vi "Begin.vi"(11 "Image Size":T1=enum."160x120") -> (0 "error out":errorcluster)   [LabVIEW 2012]
doc: "Called before other user functions, this VI is expected to open initial I/O refnums, load in file data, and do all program initialization. Notice that the <B>error out</B> terminal is simply used for data flow. Wiring it to other structures or subVIs ensures that this VI runs first."
uses:
  <vilib>/Rock Robotics/WPI/Camera/WPI_CameraImageSize.ctl
  <vilib>/Rock Robotics/SystemInterfaces/DIO/FPGA_DIOPWMChannel.ctl
  <vilib>/Rock Robotics/WPI/Camera/WPI_CameraWhite Balance Values.ctl
  <vilib>/Rock Robotics/WPI/Camera/WPI_CameraExposure Values.ctl
  <vilib>/Rock Robotics/WPI/Camera/WPI_CameraFrameRate.ctl
  <vilib>/Rock Robotics/WPI/SafetyOutput/WPI_SafetyOutputConfigMenu.ctl
  <vilib>/Rock Robotics/WPI/DriverStation/WPI_DriverStationRobotMode2.ctl
  <vilib>/Rock Robotics/WPI/Joystick/WPI_JoystickDeviceEnum.ctl
  <vilib>/Rock Robotics/WPI/Solenoid/WPI_SolenoidChannel.ctl
  <vilib>/Rock Robotics/SystemInterfaces/DIO/FPGA_DIOChannel.ctl
  <vilib>/Rock Robotics/SystemInterfaces/DIO/FPGA_DIORelayChannel.ctl
  <vilib>/Rock Robotics/SystemInterfaces/Typedef/FPGA_TypedefSolenoidModule.ctl
  <vilib>/Rock Robotics/SystemInterfaces/Typedef/FPGA_TypedefDigitalModule.ctl
  Robot Global Data.vi
  <vilib>/Rock Robotics/WPI/MotorControl/WPI_MotorControlOpen Talon.vi
  <vilib>/Rock Robotics/WPI/RobotDrive/WPI_RobotDriveOpen4MotorWithTalon.vi
  <vilib>/Rock Robotics/WPI/Solenoid/WPI_SolenoidOpenSingle.vi
  <vilib>/Rock Robotics/WPI/Compressor/WPI_CompressorGetSetRefNum.vi
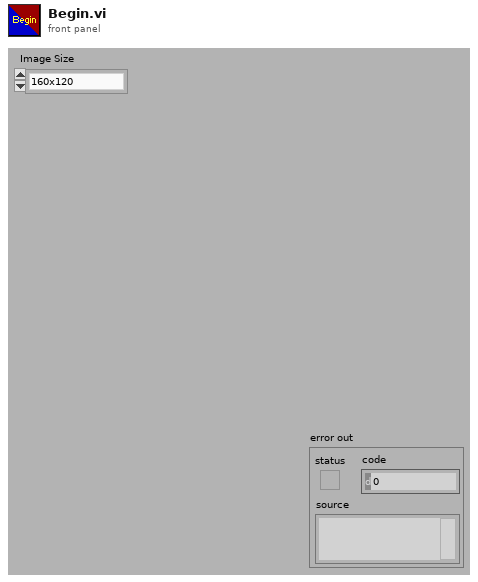
[diagram p1: front panel]
types:
  T1 = typedef "WPI_CameraImageSize.ctl" = enum16{"640x480", "320x240", "160x120"}
  T2 = typedef "WPI_SolenoidChannel.ctl" = enum8{"Solenoid 1", "Solenoid 2", "Solenoid 3", "Solenoid 4", "Solenoid 5", "Solenoid 6", "Solenoid 7", "Solenoid 8", "Invalid"}
  T3 = typedef "FPGA_TypedefSolenoidModule.ctl" = enum16{"Solenoid Module 1", "Solenoid Module 2"}
  T4 = typedef "FPGA_DIOChannel.ctl" = enum8{"DIO 1", "DIO 2", "DIO 3", "DIO 4", "DIO 5", "DIO 6", "DIO 7", "DIO 8", "DIO 9", "DIO 10", "DIO 11", "DIO 12", "DIO 13", "DIO 14", "Invalid"}
  T5 = typedef "FPGA_TypedefDigitalModule.ctl" = enum16{"Digital Module 1", "Digital Module 2"}
  T6 = typedef "FPGA_DIORelayChannel.ctl" = enum8{"Relay 1", "Relay 2", "Relay 3", "Relay 4", "Relay 5", "Relay 6", "Relay 7", "Relay 8", "Invalid"}
  T7 = typedef "FPGA_DIOPWMChannel.ctl" = enum8{"PWM 1", "PWM 2", "PWM 3", "PWM 4", "PWM 5", "PWM 6", "PWM 7", "PWM 8", "PWM 9", "PWM 10", "Invalid"}
  T8 = typedef "WPI_SafetyOutputConfigMenu.ctl" = enum16{"Enable", "Disable"}
  T9 = typedef "WPI_JoystickDeviceEnum.ctl" = enum16{"USB 1", "USB 2", "USB 3", "USB 4", "Kinect 1", "Kinect 2"}
  T10 = typedef "WPI_DriverStationRobotMode2.ctl" = enum16{"Autonomous Disabled", "Autonomous Enabled", "Teleop Disabled", "Teleop Enabled", "Timeout", "Finish", "Test Disabled", "Test Enabled"}
  T11 = typedef "WPI_CameraFrameRate.ctl" = u32
  T12 = typedef "WPI_CameraExposure Values.ctl" = enum16{"Auto", "Flicker-free 50 Hz", "Flicker-free 60 Hz", "Hold current"}
  T13 = typedef "WPI_CameraWhite Balance Values.ctl" = enum16{"Auto", "Fixed indoor", "Fixed outdoor 1", "Fixed outdoor 2", "Fixed fluorescent 1", "Fixed fluorescent 2", "Hold current"}
  T14 = typedef "WPI_DigitalOutputDevRef.ctl" = cluster{"Digital Module":T5, "DIO Channel":T4, "DevStatus":errorcluster}
  T15 = typedef "WPI_CompressorDevRef.ctl" = cluster{"DevStatus":errorcluster, "DigitalInputDevRef":T16, "RelayDevRef":T17}
  T16 = typedef "WPI_DigitalInputDevRef.ctl" = cluster{"DevStatus":errorcluster, "DIO Channel":T4, "Digital Module":T5}
  T17 = typedef "WPI_RelayDevRef.ctl" = cluster{"DevStatus":errorcluster, "Relay Channel":T6, "Digital Module":T5, "Relay Direction":T18}
  T18 = typedef "WPI_RelayDirection.ctl" = enum16{"Both directions", "Forward only", "Reverse only"}
  T19 = typedef "WPI_SolenoidDevRef.ctl" = cluster{"DevStatus":errorcluster, "Solenoid Module":T3, "Forward Solenoid Channel":T2, "Reverse Solenoid Channel":T2}
  T20 = typedef "WPI_CameraDevRef.ctl" = cluster{"Camera Address":string, "CameraStatus":errorcluster, "Acquire Image Notifier":refnum<notifier>}
  T21 = typedef "WPI_RobotDriveDevRef.ctl" = cluster{"DevStatus":errorcluster, "Motors[]":T22[], "Square Inputs":bool, "Max Output":dbl, "Isochronous":bool}
  T22 = typedef "WPI_MotorControlDeviceRef.ctl" = cluster{"DeviceStatus":errorcluster, "Type":enum16{"PWM", "CAN"}, "PWM":cluster{"Digital Module":T5, "PWM Channel":T7, "DeadBand":T23}, "CAN":cluster{"Device Number":u8, "Control Mode":T24, "Semaphore":T25, "Max Vout":dbl}, "Invert":bool, "TransformRef":T26, "InvTransformRef":T26}
  T23 = typedef "WPI_PWMDeadband.ctl" = cluster{"Name":string, "maxPositivePwm":i32, "minPositivePwm":i32, "centerPwm":i32, "maxNegativePwm":i32, "minNegativePwm":i32, "angularRange":u16}
  T24 = typedef "WPI_CANJaguar_ControlMode.ctl" = enum8{"Percent VBus", "Current", "Speed", "Position", "Voltage"}
  T25 = typedef "Semaphore RefNum" = refnum<k1>
  T26 = typedef "WPI_PWMTransform_ConPane.ctl" = refnum<vi>
  T27 = typedef "WPI_JoystickDevRef.ctl" = cluster{"Device":T9}
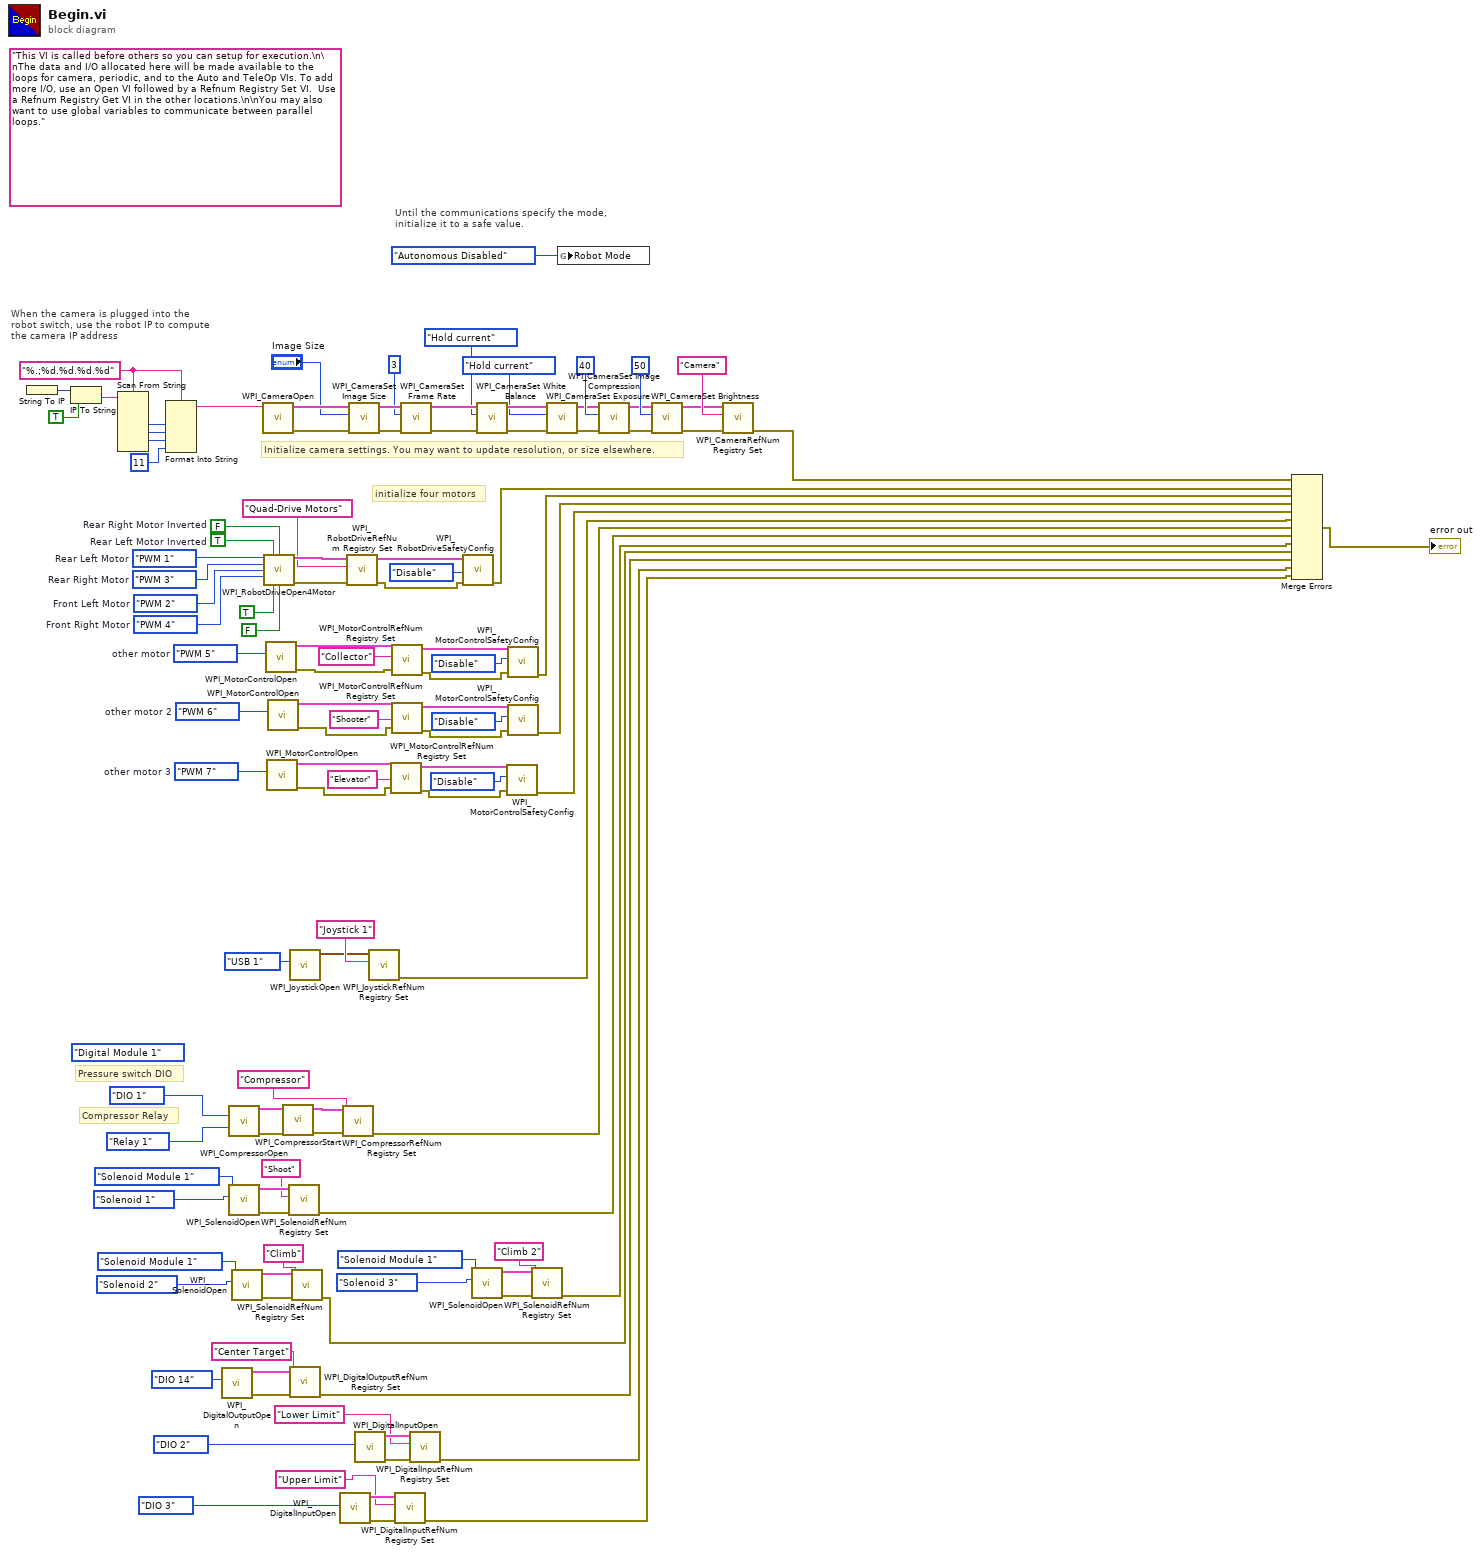
[diagram p0: block diagram]
diagram:
  (unwired) FPGA_TypedefDigitalModule."Digital Module 1" ("Pressure Switch Digital Module (Module 1)")
  w57 = FPGA_DIOPWMChannel."PWM 7"  # other motor 3
  w65 = FPGA_DIOPWMChannel."PWM 6"  # other motor 2
  w69 = FPGA_DIOPWMChannel."PWM 5"  # other motor
  w73 = FPGA_DIOPWMChannel."PWM 4"  # Front Right Motor
  w74 = FPGA_DIOPWMChannel."PWM 2"  # Front Left Motor
  w82 = "%.;%d.%d.%d.%d" ("format string")
  (unwired) "This VI is called before others so you can setup for execution.\n\nThe data and I/O allocated here will be made available to the loops for camera, periodic, and to the Auto and TeleOp VIs. To add more I/O, use an Open VI followed by a Refnum Registry Set VI.  Use a Refnum Registry Get VI in the other locations.\n\nYou may also want to use global variables to communicate between parallel loops."
  w93 = FPGA_DIOPWMChannel."PWM 3"  # Rear Right Motor
  w94 = FPGA_DIOPWMChannel."PWM 1"  # Rear Left Motor
  w116 = TRUE  # Rear Left Motor Inverted
  w117 = FALSE  # Rear Right Motor Inverted
  # "Compressor Relay"
  # "Pressure switch DIO"
  # "Until the communications specify the mode,\ninitialize it to a safe value."
  # "When the camera is plugged into the\nrobot switch, use the robot IP to compute\nthe camera IP address"
  # "initialize four motors"
  # "Initialize camera settings. You may want to update resolution, or size elsewhere."
  n1 = String To IP() -> (0:w89:u32)  [unwired: 1 in]
  n2 = IP To String(1:TRUE ("dot notation? (F)"), 2:w89) -> (0:w87:string)
  n3 = Scan From String(format string=w82, input string=w87) -> (output 1=w86:i32, output 2=w85:i32, output 3=w84:i32)  [unwired: 7 in, 3 out]
  n4 = Format Into String(format string=w82, w86, w85, w84, 11 ("Compression")) -> (resulting string=w78:string)  [unwired: 2 in, 1 out]
  n5 = call <vilib>:"WPI_DigitalOutputOpen.vi"("DIO Channel"=FPGA_DIOChannel."DIO 14") -> ("error out"=w40:errorcluster, "DigitalOutputDevRef"=w50:T14)  [unwired: 9 in]
  n6 = call <vilib>:"WPI_CompressorOpen.vi"("Pressure Switch DIO Channel"=FPGA_DIOChannel."DIO 1", "Relay Channel"=FPGA_DIORelayChannel."Relay 1") -> ("CompressorDevRef"=w36:T15, "error out"=w34:errorcluster)  [unwired: 12 in]
  n7 = call-poly <vilib>:"WPI_SolenoidOpen.vi"("Solenoid Channel"=WPI_SolenoidChannel."Solenoid 1", "Solenoid Module (Module 1)"=FPGA_TypedefSolenoidModule."Solenoid Module 1") -> ("error out"=w41:errorcluster, "SolenoidDevRef"=w53:T19)  [unwired: 8 in]
  n8 = call-poly <vilib>:"WPI_SolenoidOpen.vi"("Solenoid Channel"=WPI_SolenoidChannel."Solenoid 2", "Solenoid Module (Module 1)"=FPGA_TypedefSolenoidModule."Solenoid Module 1") -> ("error out"=w20:errorcluster, "SolenoidDevRef"=w22:T19)  [unwired: 8 in]
  n9 = call <vilib>:"WPI_CameraOpen.vi"("Camera Address"=w78) -> ("error out"=w103:errorcluster, "CameraDevRef"=w104:T20)  [unwired: 2 in, 7 out]
  n10 = call-poly <vilib>:"WPI_RobotDriveOpen4Motor.vi"("Rear Left Motor"=w94, "Rear Left Motor Inverted"=w116, "Rear Right Motor Inverted"=w117, "Rear Right Motor"=w93, "Front Left Motor"=w74, "Front Right Motor"=w73, "Front Left Motor Inverted"=TRUE, "Front Right Motor Inverted"=FALSE) -> ("RobotDriveDevRef"=w114:T21, "error out"=w112:errorcluster)  [unwired: 6 in]
  n11 = call-poly <vilib>:"WPI_MotorControlOpen.vi"("PWM Channel"=w69) -> ("error out"=w46:errorcluster, "MotorControlDeviceRef"=w72:T22)  [unwired: 9 in]
  n12 = call-poly <vilib>:"WPI_MotorControlOpen.vi"("PWM Channel"=w57) -> ("error out"=w42:errorcluster, "MotorControlDeviceRef"=w60:T22)  [unwired: 9 in]
  n13 = call-poly <vilib>:"WPI_MotorControlOpen.vi"("PWM Channel"=w65) -> ("error out"=w45:errorcluster, "MotorControlDeviceRef"=w68:T22)  [unwired: 9 in]
  n14 = call <vilib>:"WPI_CompressorStart.vi"("error in (no error)"=w34, "CompressorDevRef"=w36) -> ("error out"=w33:errorcluster, "CompressorDevRef"=w35:T15)  [unwired: 8 in]
  n15 = call <vilib>:"WPI_SolenoidRefNum Registry Set.vi"("error in (no error)"=w41, "refnum name"="Shoot", "SolenoidDevRef"=w53) -> ("error out"=w8:errorcluster)  [unwired: 7 in, 1 out]
  n16 = call <vilib>:"WPI_JoystickOpen.vi"("JoystickDevice"=WPI_JoystickDeviceEnum."USB 1") -> ("JoystickDevRef"=w76:T27)  [unwired: 10 in]
  n17 = call <vilib>:"WPI_DigitalOutputRefNum Registry Set.vi"("error in (no error)"=w40, "refnum name"="Center Target", "DigitalOutputDevRef"=w50) -> ("error out"=w7:errorcluster)  [unwired: 7 in, 1 out]
  n18 = call <vilib>:"WPI_SolenoidRefNum Registry Set.vi"("error in (no error)"=w20, "refnum name"="Climb", "SolenoidDevRef"=w22) -> ("error out"=w6:errorcluster)  [unwired: 7 in, 1 out]
  n19 = call <vilib>:"WPI_DigitalInputOpen.vi"("DIO Channel"=FPGA_DIOChannel."DIO 3") -> ("error out"=w28:errorcluster, "DigitalInputDevRef"=w27:T16)  [unwired: 9 in]
  n20 = call <vilib>:"WPI_CompressorRefNum Registry Set.vi"("error in (no error)"=w33, "refnum name"="Compressor", "CompressorDevRef"=w35) -> ("error out"=w10:errorcluster)  [unwired: 7 in, 1 out]
  n21 = call <vilib>:"WPI_RobotDriveRefNum Registry Set.vi"("error in (no error)"=w112, "refnum name"="Quad-Drive Motors", "RobotDriveDevRef"=w114) -> ("error out"=w48:errorcluster, "RobotDriveDevRef"=w81:T21)  [unwired: 7 out]
  n22 = call <vilib>:"WPI_CameraSet Image Size.vi"("error in (no error)"=w103, "Image Size"="Image Size", "CameraDevRef"=w104) -> ("error out"=w102:errorcluster, "CameraDevRef Out"=w105:T20)  [unwired: 7 out]
  n23 = call <vilib>:"WPI_DigitalInputOpen.vi"("DIO Channel"=FPGA_DIOChannel."DIO 2") -> ("error out"=w32:errorcluster, "DigitalInputDevRef"=w31:T16)  [unwired: 9 in]
  n24 = call <vilib>:"WPI_JoystickRefNum Registry Set.vi"("refnum name"="Joystick 1", "JoystickDevRef"=w76) -> ("error out"=w9:errorcluster)  [unwired: 8 in, 1 out]
  n25 = call <vilib>:"WPI_MotorControlRefNum Registry Set.vi"("error in (no error)"=w42, "refnum name"="Elevator", "MotorControlDevRef"=w60) -> ("error out"=w43:errorcluster, "MotorControlDevRef"=w59:T22)  [unwired: 7 in]
  n26 = call <vilib>:"WPI_MotorControlRefNum Registry Set.vi"("error in (no error)"=w46, "refnum name"="Collector", "MotorControlDevRef"=w72) -> ("error out"=w47:errorcluster, "MotorControlDevRef"=w71:T22)  [unwired: 7 in]
  n27 = call <vilib>:"WPI_MotorControlRefNum Registry Set.vi"("error in (no error)"=w45, "refnum name"="Shooter", "MotorControlDevRef"=w68) -> ("error out"=w44:errorcluster, "MotorControlDevRef"=w67:T22)  [unwired: 7 in]
  n28 = call <vilib>:"WPI_DigitalInputRefNum Registry Set.vi"("error in (no error)"=w28, "refnum name"="Upper Limit", "DigitalInputDevRef"=w27) -> ("error out"=w3:errorcluster)  [unwired: 7 in, 1 out]
  n29 = call <vilib>:"WPI_CameraSet Frame Rate.vi"("error in (no error)"=w102, "Frame Rate (fps)"=T11 3, "CameraDevRef"=w105) -> ("error out"=w101:errorcluster, "CameraDevRef Out"=w107:T20)  [unwired: 7 out]
  n30 = call <vilib>:"WPI_DigitalInputRefNum Registry Set.vi"("error in (no error)"=w32, "refnum name"="Lower Limit", "DigitalInputDevRef"=w31) -> ("error out"=w4:errorcluster)  [unwired: 7 in, 1 out]
  n31 = call <vilib>:"WPI_RobotDriveSafetyConfig.vi"("error in (no error)"=w48, "mode"=WPI_SafetyOutputConfigMenu."Disable", "RobotDriveDevRef"=w81) -> ("error out"=w14:errorcluster)  [unwired: 7 in, 1 out]
  n32 = call-poly <vilib>:"WPI_SolenoidOpen.vi"("Solenoid Channel"=WPI_SolenoidChannel."Solenoid 3", "Solenoid Module (Module 1)"=FPGA_TypedefSolenoidModule."Solenoid Module 1") -> ("error out"=w15:errorcluster, "SolenoidDevRef"=w17:T19)  [unwired: 8 in]
  n33 = call <vilib>:"WPI_CameraSet White Balance.vi"("error in (no error)"=w101, "White Balance"=WPI_CameraWhite_Balance_Values."Hold current", "CameraDevRef"=w107) -> ("error out"=w100:errorcluster, "CameraDevRef Out"=w106:T20)  [unwired: 7 out]
  n34 = call <vilib>:"WPI_MotorControlSafetyConfig.vi"("error in (no error)"=w43, "mode"=WPI_SafetyOutputConfigMenu."Disable", "MotorControlDevRef"=w59) -> ("error out"=w11:errorcluster)  [unwired: 7 in, 1 out]
  n35 = call <vilib>:"WPI_MotorControlSafetyConfig.vi"("error in (no error)"=w47, "mode"=WPI_SafetyOutputConfigMenu."Disable", "MotorControlDevRef"=w71) -> ("error out"=w13:errorcluster)  [unwired: 7 in, 1 out]
  n36 = call <vilib>:"WPI_MotorControlSafetyConfig.vi"("error in (no error)"=w44, "mode"=WPI_SafetyOutputConfigMenu."Disable", "MotorControlDevRef"=w67) -> ("error out"=w12:errorcluster)  [unwired: 7 in, 1 out]
  n37 = call <vilib>:"WPI_SolenoidRefNum Registry Set.vi"("error in (no error)"=w15, "refnum name"="Climb 2", "SolenoidDevRef"=w17) -> ("error out"=w5:errorcluster)  [unwired: 7 in, 1 out]
  n38 = call <vilib>:"WPI_CameraSet Exposure.vi"("error in (no error)"=w100, "Exposure"=WPI_CameraExposure_Values."Hold current", "CameraDevRef"=w106) -> ("error out"=w99:errorcluster, "CameraDevRef Out"=w109:T20)  [unwired: 7 out]
  n39 = global write "Robot Global Data.vi" "Robot Mode"(WPI_DriverStationRobotMode2."Autonomous Disabled" ("Robot Mode")) -> ()
  n40 = call <vilib>:"WPI_CameraSet Image Compression.vi"("error in (no error)"=w99, "Compression"=40, "CameraDevRef"=w109) -> ("error out"=w98:errorcluster, "CameraDevRef Out"=w108:T20)  [unwired: 7 out]
  n41 = call <vilib>:"WPI_CameraSet Brightness.vi"("error in (no error)"=w98, "Brightness"=50, "CameraDevRef"=w108) -> ("error out"=w96:errorcluster, "CameraDevRef Out"=w97:T20)  [unwired: 7 out]
  n42 = call <vilib>:"WPI_CameraRefNum Registry Set.vi"("error in (no error)"=w96, "refnum name"="Camera", "CameraDevRef"=w97) -> ("error out"=w2:errorcluster)  [unwired: 8 out]
  n43 = Merge Errors(w2, w14, w13, w12, w11, w9, w10, w8, w5, w6, w7, w4, w3) -> (→"error out":errorcluster)
